vi "setStepNLoopParams.vi"(0 "MultiAxisController in":refnum<class "_MultiAxisController.lvclass">, 2 "axis":T1, 3 "set_params?":T3, 4 "step_n_params":T2, 5 "error in (no error)":errorcluster) -> (14 "MultiAxisController out":refnum<class "_MultiAxisController.lvclass">, 17 "success?":bool, 18 "response":string, 19 "error out":errorcluster)   [LabVIEW 2020, in "classes.lvlib" / "_MultiAxisController.lvclass"]
doc: "Produced By:\n\n<B>Kod Integrations, LLC</B>\n4835 Marianne Drive\nMount Airy, MD 21771\nhttp://www.kodintegrations.com\nemail: info@kodintegrations.com\nphone: (240) 687-1288"
uses:
  _MultiAxisController.lvclass
  Controller/_Controller.lvclass
  C:/GEECS/Developers Version/source/Device Drivers/Newmark-NSC-A/Arcus Driver 3.0.0/ArcusUsbComm/classes/Controller/_Controller.lvclass
  C:/GEECS/Developers Version/source/Device Drivers/Newmark-NSC-A/Arcus Driver 3.0.0/ArcusUsbComm/classes/MultiAxisController/_MultiAxisController.lvclass
  common/controls/axis.ctl
  libraries/common.lvlib
  common/controls/step_n_loop_params_write_logic.ctl
  common/controls/step_n_params.ctl
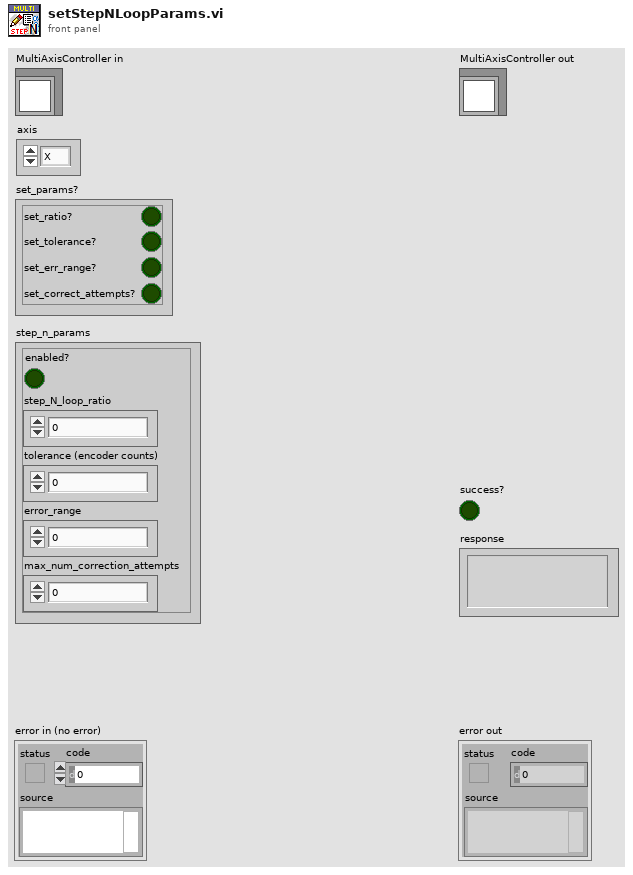
[diagram p1: front panel]
types:
  T1 = typedef "common.lvlib/axis.ctl" = enum16{"X", "Y", "Z", "U"}
  T2 = typedef "common.lvlib/step_n_params.ctl" = cluster{"step_N_loop_ratio":dbl, "tolerance (encoder counts)":u32, "error_range":i32, "max_num_correction_attempts":i32, "enabled?":bool}
  T3 = typedef "common.lvlib/step_n_loop_params_write_logic.ctl" = cluster{"set_ratio?":bool, "set_tolerance?":bool, "set_err_range?":bool, "set_correct_attempts?":bool}
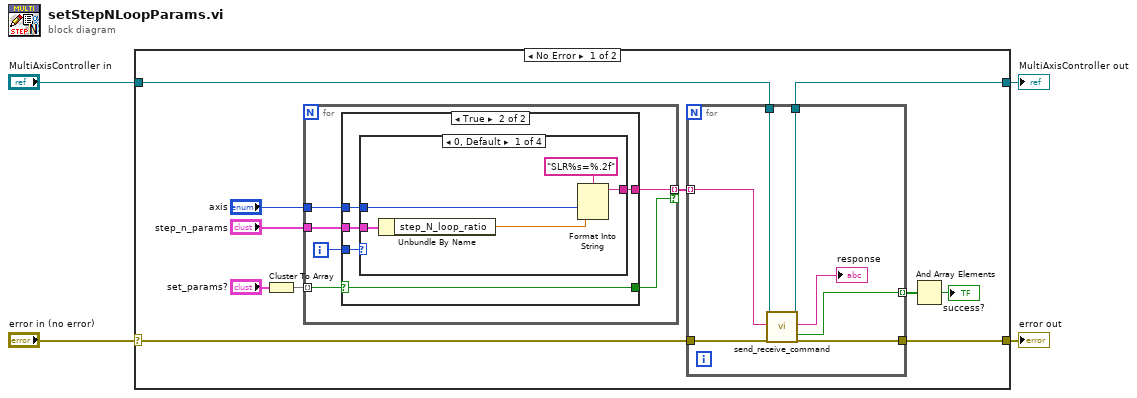
[diagram p0: block diagram]
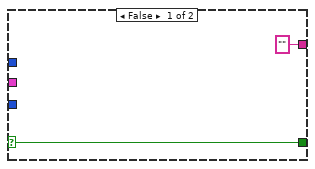
[diagram p2: hidden frame]
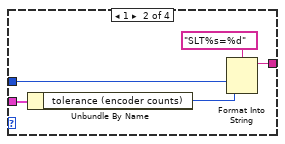
[diagram p3: hidden frame]
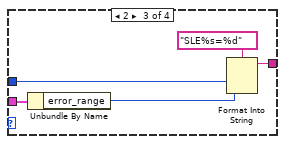
[diagram p4: hidden frame]
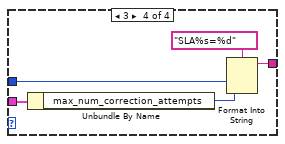
[diagram p5: hidden frame]
diagram:
  n1 = case shown="No Error" "error in (no error)" {
    selector: "error in (no error)" -> [w10 w57]
    tunnel: [w9 w57] -> w3
    tunnel: [w7 w56] -> w1
    tunnel: "MultiAxisController in" -> [w8 w56]
    frame No Error {
      n2 = Cluster To Array(cluster="set_params?") -> (array=w12:bool[])
      n3 = for {
        tunnel: "axis" -> [w20]
        tunnel: "step_n_params" -> [w19]
        tunnel: w12 -> [w18] mode=indexing
        tunnel: [w17] -> w11 mode=indexing if=w16
        i -> [w21]
        n4 = case shown="True" w18 {
          selector: w18 -> [w22 w24]
          tunnel: w21 -> [_ w28]
          tunnel: w20 -> [_ w27]
          tunnel: w19 -> [_ w26]
          tunnel: ["" w25] -> w17
          tunnel: [w22 w24] -> w16
          frame False {
          }
          frame True {
            n5 = case shown="0, Default" w28 {
              tunnel: w27 -> [w32 w37 w42 w47]
              tunnel: w26 -> [w31 w36 w41 w46]
              tunnel: [w29 w34 w39 w44] -> w25
              frame 0, Default {
                n6 = Unbundle By Name(w31) -> ("step_N_loop_ratio"=w30:dbl)
                n7 = Format Into String(format string="SLR%s=%.2f", w32, w30) -> (resulting string=w29:string)  [unwired: 2 in, 1 out]
              }
              frame 1 {
                n8 = Unbundle By Name(w36) -> ("tolerance (encoder counts)"=w35:u32)
                n9 = Format Into String(format string="SLT%s=%d", w37, w35) -> (resulting string=w34:string)  [unwired: 2 in, 1 out]
              }
              frame 2 {
                n10 = Unbundle By Name(w41) -> ("error_range"=w40:i32)
                n11 = Format Into String(format string="SLE%s=%d", w42, w40) -> (resulting string=w39:string)  [unwired: 2 in, 1 out]
              }
              frame 3 {
                n12 = Unbundle By Name(w46) -> ("max_num_correction_attempts"=w45:i32)
                n13 = Format Into String(format string="SLA%s=%d", w47, w45) -> (resulting string=w44:string)  [unwired: 2 in, 1 out]
              }
            }
          }
        }
      }
      n14 = for {
        tunnel: w10 -> [w55]
        tunnel: [w54] -> w9
        tunnel: w8 -> [w53]
        tunnel: [w52] -> w7
        tunnel: w11 -> [w51] mode=indexing
        tunnel: [w50] -> w6 mode=indexing
        n15 = call "send_receive_command.vi"("reference (in)"=w53, "ASCII Command (in)"=w51, "error in (no error)"=w55) -> ("reference (out)"=w52:refnum<class "_MultiAxisController.lvclass">, "response (out)"=→"response":string, "success?"=w50:bool, "error out"=w54:errorcluster)  [unwired: 12 in, 1 out]
      }
      n16 = And Array Elements(Boolean array=w6) -> (logical AND=→"success?":bool)
    }
    frame Error {
    }
  }
  "error out" <- w3
  "MultiAxisController out" <- w1
